vi "SamplePositionToImage (SubVI).vi"(4 "sample_y":fxp<+/-,26,5>, 5 "image size_y":u16, 6 "sample_x":fxp<+/-,26,5>, 7 "image size_x":u16, 8 "sample end_y":fxp<+/-,26,5>, 9 "sample end_x":fxp<+/-,26,5>, 10 "sample start_y":fxp<+/-,26,5>, 11 "sample start_x":fxp<+/-,26,5>) -> (0 "image_y":u16, 1 "image_x":u16, 2 "increment_y":fxp<+/-,43,6>, 3 "increment_x":fxp<+/-,43,6>)   [LabVIEW 2017]
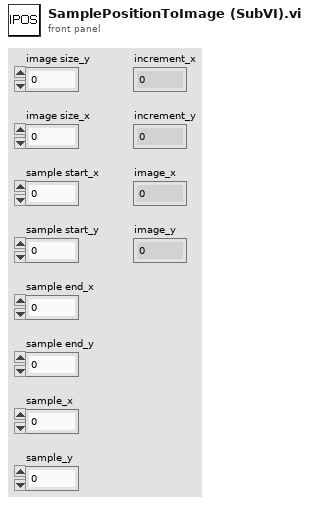
[diagram p1: front panel]
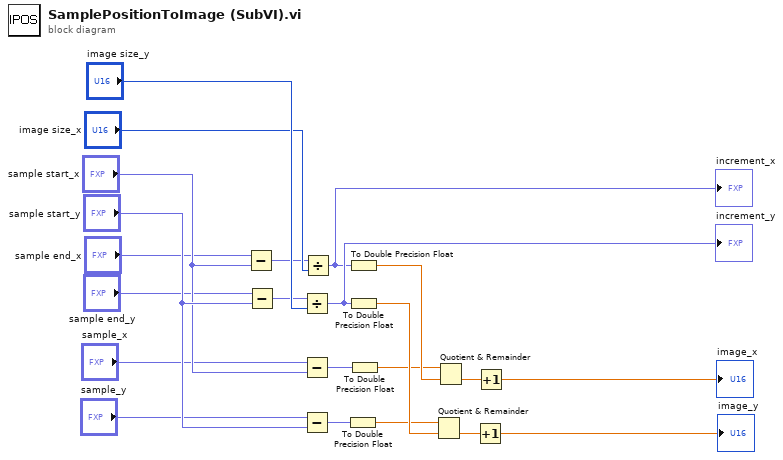
[diagram p0: block diagram]
diagram:
  n1 = Subtract(x="sample end_x", y="sample start_x") -> (x-y=w2:fxp<+/-,27,6>)
  n2 = Subtract(x="sample end_y", y="sample start_y") -> (x-y=w5:fxp<+/-,27,6>)
  n3 = Divide(x=w5, y="image size_y") -> (x/y=w20:fxp<+/-,43,6>)
  "increment_y" <- w20
  n4 = Subtract(x="sample_x", y="sample start_x") -> (x-y=w11:fxp<+/-,27,6>)
  n5 = Subtract(x="sample_y", y="sample start_y") -> (x-y=w13:fxp<+/-,27,6>)
  n6 = Divide(x=w2, y="image size_x") -> (x/y=w19:fxp<+/-,43,6>)
  "increment_x" <- w19
  n7 = To Double Precision Float(number=w13) -> (double precision float=w14:dbl)
  n8 = To Double Precision Float(number=w19) -> (double precision float=w15:dbl)
  n9 = To Double Precision Float(number=w20) -> (double precision float=w16:dbl)
  n10 = To Double Precision Float(number=w11) -> (double precision float=w12:dbl)
  n11 = Quotient & Remainder(x=w14, y=w16) -> (floor(x/y)=w18:dbl)  [unwired: 1 out]
  n12 = Quotient & Remainder(x=w12, y=w15) -> (floor(x/y)=w17:dbl)  [unwired: 1 out]
  n13 = Increment(x=w18) -> (x+1=→"image_y":dbl)
  n14 = Increment(x=w17) -> (x+1=→"image_x":dbl)
